vi "Menu Act Preferences.vi"(8 "error in (no error)":errorcluster, 11 "LF2R IDE in":refnum<class "Main Panel.lvclass">) -> (0 "error out":errorcluster, 3 "LF2R IDE out":refnum<class "Main Panel.lvclass">)   [LabVIEW 2018, in "Main Panel.lvlib" / "Main Panel.lvclass"]
uses:
  Main Panel.lvclass
  C:/Program Files (x86)/National Instruments/LabVIEW 2018/vi.lib/MGI/Panel Manager/Panel Actor/Panel Actor/Panel Actor.lvclass
  Configuration Window/Configuration Window/Configuration Window.lvclass
  Main Panel.lvclass/Main Panel.ctl
  Configuration Window/Configuration Window/Configuration Window.lvclass/Configuration Window.ctl
  Configuration Window/Configuration Window/Write Configuration.vi
  <vilib>/MGI/Panel Manager/Panel/Panel/Window/Dialog/Dialog.lvclass
  C:/Program Files (x86)/National Instruments/LabVIEW 2018/vi.lib/MGI/Panel Manager/Panel/Panel/Panel.lvclass
  <vilib>/MGI/Panel Manager/Panel/Panel/Window/Dialog/Dialog.vi
  <vilib>/MGI/Panel Manager/Panel Actor/Panel Actor/Panel Actor.lvclass
  <vilib>/MGI/Panel Manager/Panel/Panel.lvlib
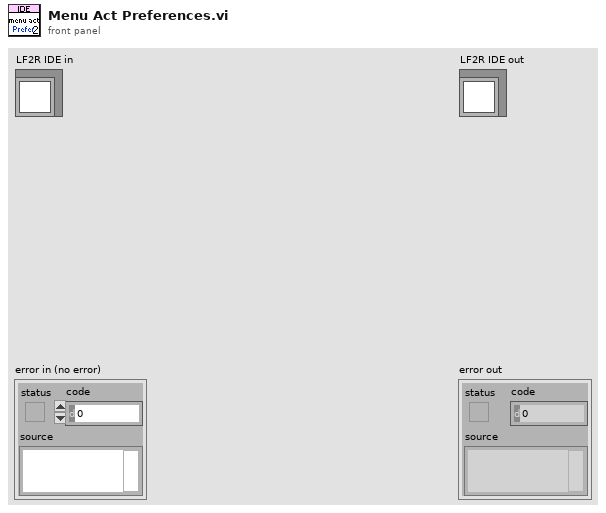
[diagram p1: front panel]
types:
  T1 = typedef "Main Panel.lvlib/Main Panel.lvclass/Const Configuration.ctl" = cluster{"Language":cluster{"Name":string}, "Path Config":T2, "Image Viewer Config":T3}
  T2 = typedef "Main Panel.lvlib/Main Panel.lvclass/Const Path Setting.ctl" = cluster{"Data Folder Path":path, "PNG Folder Path":path, "mp3 Folder Path":path}
  T3 = typedef "Main Panel.lvlib/Main Panel.lvclass/Const Image Viewer Setting.ctl" = cluster{"Center Point":cluster{"Size":i32, "Color":u32, "Show?":bool}, "bp Point":cluster{"Size":i32, "Color":u32, "Show?":bool}, "w Point":cluster{"Size":i32, "Color":u32, "Show?":bool}, "b Box":cluster{"Fill Color":u32, "Border Color":u32, "Show?":bool}, "i Box":cluster{"Fill Color":u32, "Border Color":u32, "Show?":bool}, "o Point":cluster{"Size":i32, "Color":u32, "Show?":bool}, "c Point":cluster{"Size":i32, "Color":u32, "Show?":bool}}
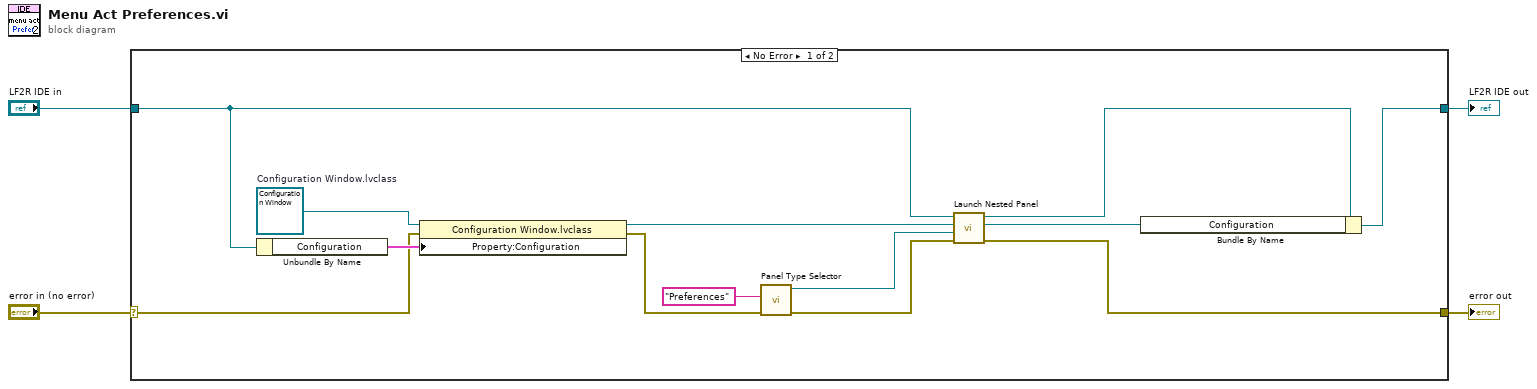
[diagram p0: block diagram]
diagram:
  n1 = case shown="No Error" "error in (no error)" {
    selector: "error in (no error)" -> [w5 w19]
    tunnel: [w14 w19] -> w3
    tunnel: [w12 w18] -> w1
    tunnel: "LF2R IDE in" -> [w7 w18]
    frame No Error {
      w17 = refnum<class "Configuration Window.lvclass"> refnum  # Configuration Window.lvclass
      n2 = Unbundle By Name(w7) -> ("Configuration"=w6:T1)
      n3 = property class="Configuration Window.lvclass"(reference=w17, error in=w5, "Property:Configuration"=w6) -> (reference out=w9:refnum<class "Configuration Window.lvclass">, error out=w8:errorcluster)
      n4 = call-poly <vilib>:"Panel Type Selector.vi"("Error In"=w8, "Default Title"="Preferences") -> ("Error Out"=w10:errorcluster, "Dialog out"=w16:refnum<class "Dialog.lvclass">)  [unwired: 8 in]
      n5 = call <vilib>:"Launch Nested Panel.vi"("error in (no error)"=w10, "Panel"=w16, "Nested Panel Actor"=w9, "Panel Actor in"=w7) -> ("error out"=w14:errorcluster, "Nested Actor's Enqueuer"=w11:refnum<class "Message Enqueuer.lvclass">, "Panel Actor out"=w13:refnum<class "Main Panel.lvclass">)  [unwired: 4 in, 1 out]
      n6 = Bundle By Name(cluster=w13, "Configuration"=w11) -> (w12:refnum<class "Main Panel.lvclass">)
    }
    frame Error {
    }
  }
  "error out" <- w3
  "LF2R IDE out" <- w1
